vi "Copy StartSync.vi"(8 "error in (no error)":errorcluster, 11 "project folder":path) -> (0 "error out":errorcluster, 3 "project folder out":path)   [LabVIEW 2019]
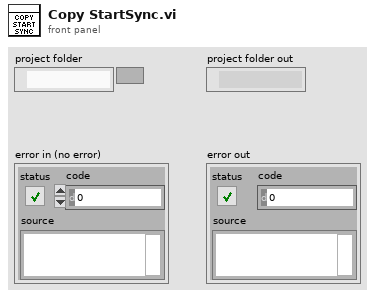
[diagram p1: front panel]
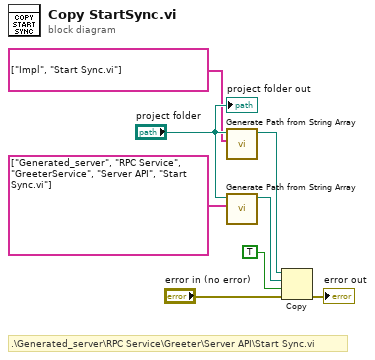
[diagram p0: block diagram]
diagram:
  # ".\\Generated_server\\RPC Service\\Greeter\\Server API\\Start Sync.vi"
  n1 = call "Generate Path from String Array.vi"("String Array"=string[] ["Impl", "Start Sync.vi"], "Base Path"="project folder") -> ("project folder out"=w1:path)  [unwired: 9 in]
  n2 = call "Generate Path from String Array.vi"("String Array"=string[] ["Generated_server", "RPC Service", "GreeterService", "Server API", "Start Sync.vi"], "Base Path"="project folder") -> ("project folder out"=w5:path)  [unwired: 9 in]
  n3 = Copy(8:"error in (no error)", 9:TRUE ("overwrite (F)"), 10:w5, 11:w1) -> (0:→"error out":errorcluster)  [unwired: 1 in, 2 out]
  "project folder out" <- "project folder"
